vi "Info to Map.vi"(6 "File Size (kB)":i32, 8 "error in (no error)":errorcluster, 9 "Release Notes":string, 10 "Library Description":string, 11 "NIPKG Inputs":T1) -> (0 "error out":errorcluster, 2 "Map":map{string, string}(c390))   [LabVIEW 2019, in "NIPKG Packager.lvclass"]
uses:
  NIPKG Packager.lvclass
  NIPKG Inputs.ctl
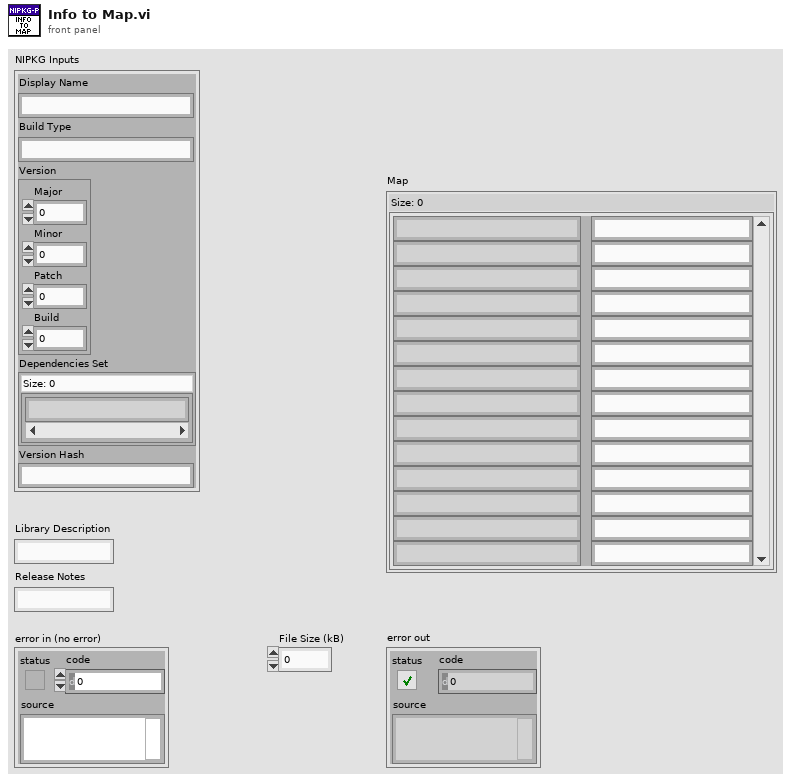
[diagram p1: front panel]
types:
  T1 = typedef "NIPKG Packager.lvclass/NIPKG Inputs.ctl" = cluster{"Display Name":string, "Build Type":string, "Version":cluster{"Major":i32, "Minor":i32, "Patch":i32, "Build":i32}, "Dependencies Set":set{string}, "Version Hash":string}
  T2 = cluster{"Major":i32, "Minor":i32, "Patch":i32, "Build":i32}
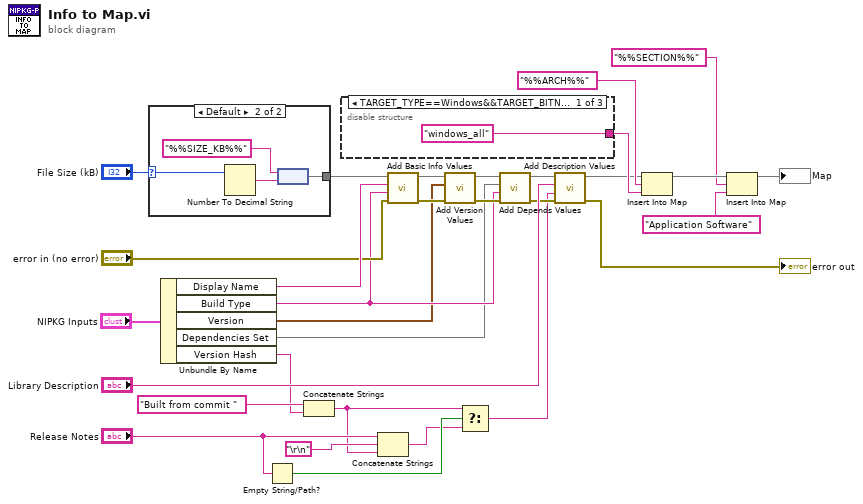
[diagram p0: block diagram]
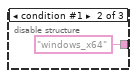
[diagram p3: hidden frame]
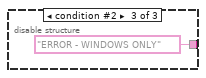
[diagram p4: hidden frame]
diagram:
  n1 = case shown="Default" "File Size (kB)" {
    selector: "File Size (kB)" -> [_ w34]
    tunnel: [_ w32] -> w27
    frame 0 {
      # "Size is not a required attribute"
    }
    frame Default {
      n2 = Number To Decimal String(number=w34) -> (decimal integer string=w33:string)  [unwired: 1 in]
      n3 = node("%%SIZE_KB%%" ("key"), w33) -> (w32:map{string, string})
    }
  }
  n4 = Unbundle By Name("NIPKG Inputs") -> ("Display Name"=w12:string, "Build Type"=w10:string, "Version"=w9:T2, "Dependencies Set"=w8:set{string}, "Version Hash"=w4:string)
  n5 = Empty String/Path?(string/path="Release Notes") -> (empty?=w6:bool)
  n6 = Concatenate Strings("Built from commit " ("string"), w4) -> (w3:string)
  n7 = disable-structure shown="TARGET_TYPE==Windows&&TARGET_BITNESS==32" {
    disable-tunnel: ["windows_all" ("value") "windows_x64" ("value") "ERROR - WINDOWS ONLY" ("value")] -> w29
    frame condition #0 (active) {
    }
    frame condition #1 {
    }
    frame condition #2 {
    }
  }
  n8 = Concatenate Strings("Release Notes", "\r\n", w3) -> (w2:string)
  n9 = call "Add Basic Info Values.vi"("error in (no error)"="error in (no error)", "Build Type String"=w10, "LVLIB Name"=w12, "Map in"=w27) -> ("error out"=w26:errorcluster, "Map out"=w25:map{string, string})  [unwired: 6 in]
  n10 = call "Add Version Values.vi"("error in (no error)"=w26, "Version"=w9, "Map in"=w25) -> ("error out"=w18:errorcluster, "Map out"=w28:map{string, string})  [unwired: 7 in]
  n11 = Select(t=w3, s=w6, f=w2) -> (s? t:f=w1:string)
  n12 = call "Add Depends Values.vi"("error in (no error)"=w18, "Build Type String"=w10, "Dependencies Set"=w8, "Map in"=w28) -> ("error out"=w19:errorcluster, "Map out"=w24:map{string, string})  [unwired: 6 in]
  n13 = call "Add Description Values.vi"("error in (no error)"=w19, "Release Notes"=w1, "Description"="Library Description", "Map in"=w24) -> ("error out"=→"error out":errorcluster, "Map out"=w23:map{string, string})  [unwired: 6 in]
  n14 = Insert Into Map(map in=w23, key="%%ARCH%%", value=w29) -> (map out=w17:map{string, string})  [unwired: 2 out]
  n15 = Insert Into Map(map in=w17, key="%%SECTION%%", value="Application Software") -> (map out=→"Map":map{string, string})  [unwired: 2 out]
